vi "NI VeriStand - Get Model Execution State.vi"(8 "error in (no error)":errorcluster, 11 "Model in":T2) -> (0 "error out":errorcluster, 1 "Model Time":dbl, 2 "Model State":T1 items=["Running", "Paused", "Resetting", "Idle", "Stopped"], 3 "Model out":T2)   [LabVIEW 2020, in "NI_VS Model ExecutionAPI.lvlib"]
doc: "Returns the state and running time of the model you specify."
uses:
  <vilib>/NI VeriStand/Execution/Model/NI_VS Model ExecutionAPI.lvlib
  <vilib>/NI VeriStand/Execution/Model/ModelAPI.ctl
  NationalInstruments.VeriStand.ClientAPI
  <vilib>/NI VeriStand/Execution/Model/ModelState.ctl
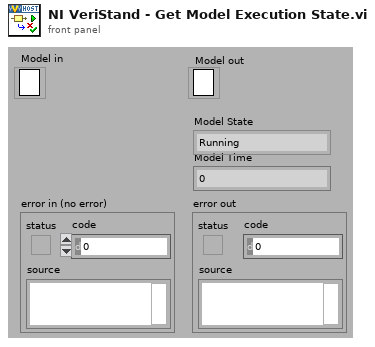
[diagram p1: front panel]
types:
  T1 = typedef "NI_VS Model ExecutionAPI.lvlib/ModelState.ctl" = u8
  T2 = typedef "NI_VS Model ExecutionAPI.lvlib/ModelAPI.ctl" = refnum<k24>
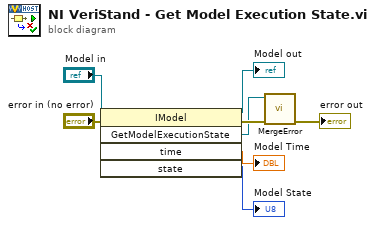
[diagram p0: block diagram]
diagram:
  n1 = invoke class="IModel" method="GetModelExecutionState"(reference="Model in", error in="error in (no error)") -> (reference out=→"Model out":T2, error out=w6:errorcluster, "GetModelExecutionState"=w5:refnum<k24>, "time"=→"Model Time":dbl, "state"=→"Model State":u8)  [unwired: 3 in]
  n2 = call <vilib>:"MergeError.vi"("error in (no error)"=w6, "Error"=w5) -> ("error out"=→"error out":errorcluster)  [unwired: 9 out]
